vi "onProcessKilled.vi"(11 "SMO.ErrorInjection in":refnum<class "SMO.ErrorInjection.lvclass">) -> ()   [LabVIEW 2013, in "SMO.ErrorInjection.lvclass"]
uses:
  SMO.ErrorInjection.lvclass
  src/SMO/SMO.lvclass
panel:
  # "This method is called if the call chain of the SMO\nis leaving memory while the process is running.\nAssume all references created in caller's thread to\nbe invalid."
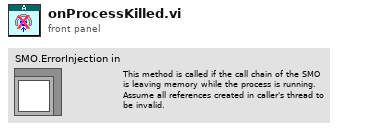
[diagram p1: front panel]
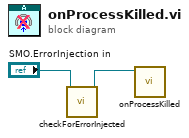
[diagram p0: block diagram]
diagram:
  n1 = call "checkForErrorInjected.vi"("SMO.ErrorInjection in"="SMO.ErrorInjection in") -> ("SMO.ErrorInjection dup"=w1:refnum<class "SMO.ErrorInjection.lvclass">)  [unwired: 9 in, 1 out]
  n2 = call-parent "onProcessKilled.vi"("SMO in"=w1) -> ()  [unwired: 11 in]
